vi "Read Message.vi"(8 "error in (no error)":errorcluster, 9 "timeout in ms (-1)":i32=-1, 11 "WebSocket Connection in":refnum<class "WebSocket Connection.lvclass">) -> (0 "error out":errorcluster, 1 "timed out?":bool, 2 "message":string, 3 "WebSocket Connection out":refnum<class "WebSocket Connection.lvclass">, 4 "binary?":bool)   [LabVIEW 2019, in "WebSocket Server Toolkit.lvlib" / "WebSocket Connection.lvclass"]
doc: "<b>Description</b> Read a message from the WebSocket connection.\n\n<b>Inputs</b>\n<b>timeout</b>: The number of milliseconds to wait for a new message.\n\n<b>Outputs</b>\n<b>binary</b>: TRUE if the client indicated that the message contains binary data.\n<b>timed out?</b>: Whether this operation timed out while waiting for a message.\n<b>message</b>: The received message."
uses:
  WebSocket Connection.lvclass
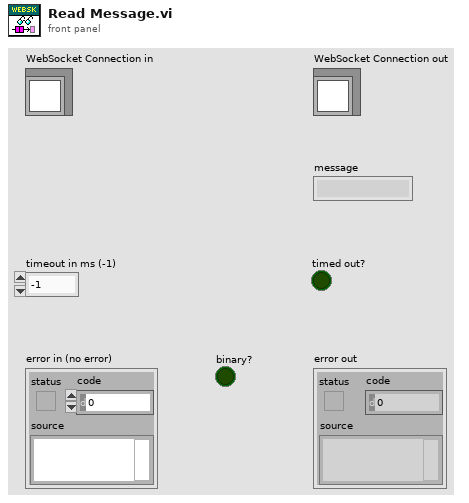
[diagram p1: front panel]
types:
  T1 = typedef "WebSocket Server Toolkit.lvlib/frame_data.ctl" = cluster{"binary?":bool, "frames":string[]}
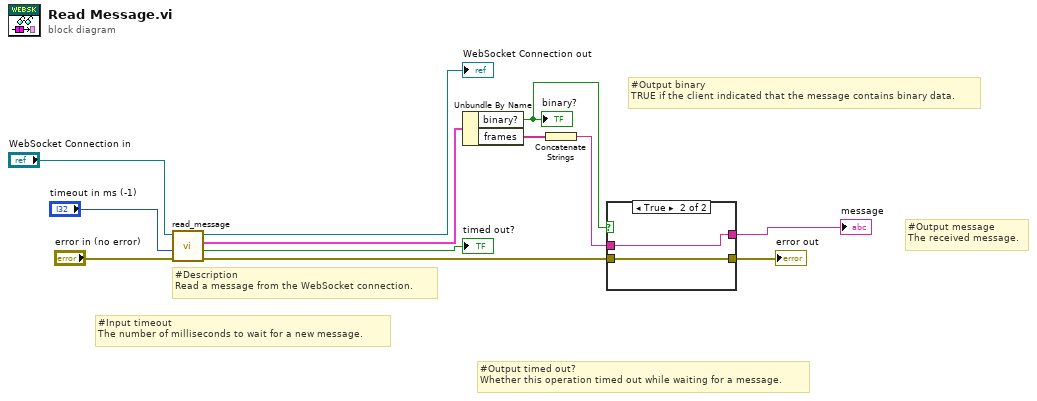
[diagram p0: block diagram]
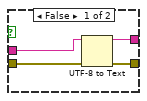
[diagram p2: hidden frame]
diagram:
  # "#Output binary\nTRUE if the client indicated that the message contains binary data."
  # "#Output timed out?\nWhether this operation timed out while waiting for a message."
  # "#Output message\nThe received message."
  # "#Input timeout\nThe number of milliseconds to wait for a new message."
  # "#Description\nRead a message from the WebSocket connection."
  n1 = call-dynamic "read_message.vi"("error in (no error)"="error in (no error)", "timeout in ms (-1)"="timeout in ms (-1)", "WebSocket Connection in"="WebSocket Connection in") -> ("error out"=w2:errorcluster, "timed out?"=→"timed out?":bool, "element"=w7:T1, "WebSocket Connection out"=→"WebSocket Connection out":refnum<class "WebSocket Connection.lvclass">)  [unwired: 5 in]
  n2 = Unbundle By Name(w7) -> ("binary?"=w5:bool, "frames"=w6:string[])
  "binary?" <- w5
  n3 = Concatenate Strings(w6) -> (w4:string)
  n4 = case shown="True" w5 {
    tunnel: w4 -> [w16 w18]
    tunnel: [w15 w18] -> w3
    tunnel: [w14 w17] -> w1
    tunnel: w2 -> [w13 w17]
    frame False {
      n5 = UTF-8 to Text(8:w13, 11:w16) -> (0:w14:errorcluster, 3:w15:string)  [unwired: 1 in]
    }
    frame True {
    }
  }
  "error out" <- w1
  "message" <- w3
